vi "Decode Balls.vi"(8 "error in":errorcluster, 9 "array":u8[](array[numeric]), 10 "Key":i32=5) -> (0 "error out":errorcluster, 1 "array w/ subset deleted out":u8[](array[numeric]), 3 "Array":T1[](array[typedef]))   [LabVIEW 2016]
uses:
  SSL Detection Ball.ctl
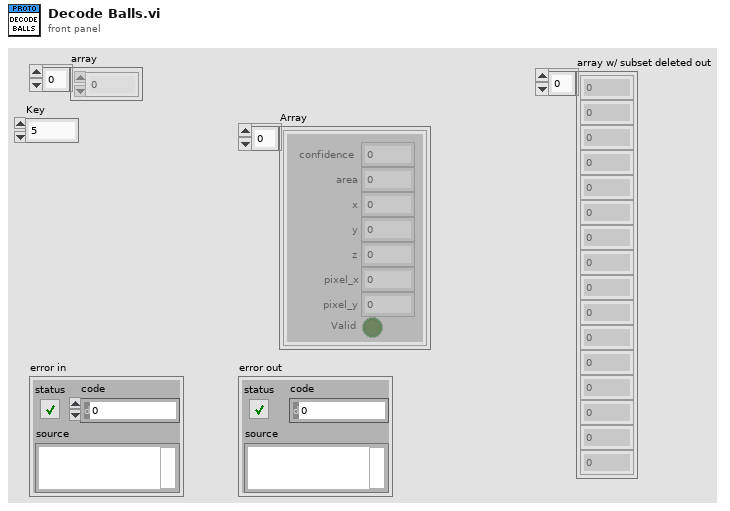
[diagram p1: front panel]
types:
  T1 = typedef "SSL Detection Ball.ctl" = cluster{"x":sgl, "area":u32, "confidence":sgl, "y":sgl, "z":sgl, "pixel_x":sgl, "pixel_y":sgl, "Valid":bool}
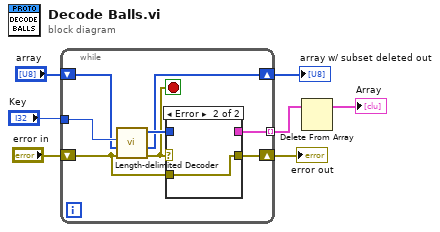
[diagram p0: block diagram]
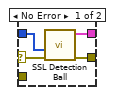
[diagram p2: hidden frame]
diagram:
  n1 = while {
    shift-right: [w12] -> w4
    shift-left: "array" -> [w8]
    tunnel: [w15] -> w3 mode=indexing
    shift-right: [w14] -> w6
    shift-left: "error in" -> [w11]
    tunnel: "Key" -> [w9]
    stop <- w10 stop-if-true
    n2 = call "Length-delimited Decoder.vi"("error in (no error)"=w11, "Array"=w8, "Key"=w9) -> ("error out"=w10:errorcluster, "array w/ subset deleted"=w12:u8[], "Length-delimited"=w13:u8[])  [unwired: 5 in, 1 out]
    n3 = case shown="Error" w10 {
      selector: w10 -> [w17 _]
      tunnel: [w19 _] -> w15
      tunnel: [w18 w20] -> w14
      tunnel: w13 -> [w16 _]
      tunnel: w11 -> [_ w20]
      frame No Error {
        n4 = call "SSL Detection Ball.vi"("error in"=w17, "Array"=w16) -> ("error out"=w18:errorcluster, "Detection Ball"=w19:T1)  [unwired: 7 in, 1 out]
      }
      frame Error {
      }
    }
  }
  "error out" <- w6
  "array w/ subset deleted out" <- w4
  n5 = Delete From Array(array=w3) -> (array with subset deleted=→"Array":T1[])  [unwired: 2 in, 1 out]
